vi "Formate Assertions for Description.vi"(7 "Style":enum16{"Diff", "Plain"}(ring), 10 "Item":string, 11 "Result Model In":refnum<class "Result Model.lvclass">) -> (2 "Assertions Description":string)   [LabVIEW 2020, in "Result Model.lvclass"]
uses:
  Result Model.lvclass
  Result Model.lvclass/Result Model.ctl
  Framework/Utilities/Utilities.lvlib
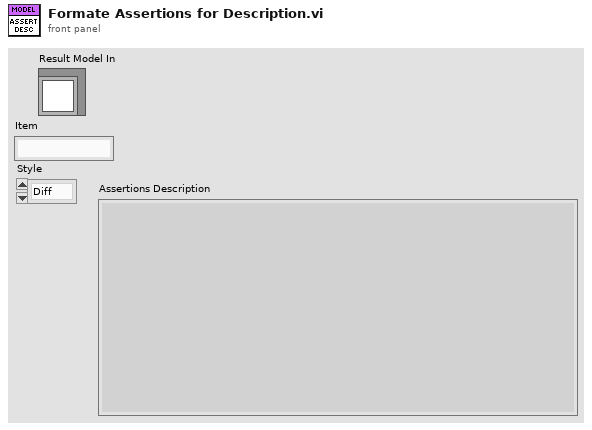
[diagram p1: front panel]
types:
  T1 = typedef "Result.lvlib/Type.ctl" = enum16{"Test Case", "Test Suite", "Test Run", "Pass", "Fail", "Skip", "Pass if", "Fail if", "Pass if Error", "Fail if Error", "Pass if Equal", "Fail if Equal"}
  T2 = typedef "Result.lvlib/Status.ctl" = enum16{"", "Passed", "Failed", "Error", "Skipped", "Setup Error", "Broken", "Teardown Error"}
  T3 = map{string, cluster{"Result Type":T1, "Status":T2, "Description":string, "Data":cluster{"Expected":variant, "Actual":variant, "Delta":variant}}[]}
  T4 = cluster{"Result Type":T1, "Status":T2, "Description":string, "Data":cluster{"Expected":variant, "Actual":variant, "Delta":variant}}[]
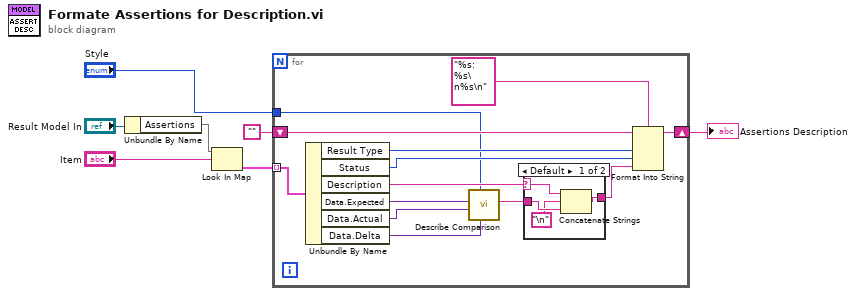
[diagram p0: block diagram]
diagram:
  n1 = Unbundle By Name("Result Model In") -> ("Assertions"=w4:T3)
  n2 = Look In Map(map=w4, key="Item") -> (value=w6:T4)  [unwired: 1 in, 1 out]
  n3 = for {
    tunnel: w6 -> [w19] mode=indexing
    shift-right: [w14] -> w2
    shift-left: "" -> [w15]
    tunnel: "Style" -> [w8]
    n4 = Unbundle By Name(w19) -> ("Result Type"=w12:T1, "Status"=w11:T2, "Description"=w9:string, "Data.Expected"=w18:variant, "Data.Actual"=w17:variant, "Data.Delta"=w16:variant)
    n5 = call "Describe Comparison.vi"("Delta"=w16, "Style"=w8, "Actual"=w17, "Expected"=w18) -> ("Description"=w13:string)  [unwired: 7 in]
    n6 = case shown="Default" w9 {
      selector: w9 -> [w23 _]
      tunnel: w13 -> [w22 w25]
      tunnel: [w24 w25] -> w10
      frame Default {
        n7 = Concatenate Strings(w23, "\n", w22) -> (w24:string)
      }
      frame "" {
      }
    }
    n8 = Format Into String(format string="%s: %s\n%s\n", initial string=w15, w12, w11, w10) -> (resulting string=w14:string)  [unwired: 1 in, 1 out]
  }
  "Assertions Description" <- w2
